vi "FastOffset.vi"() -> ()   [LabVIEW 2011]
panel:
  out "OffDEC_dir":string
  in  "Offset RA":dbl=-30.0 caption="A.D." format="%.2f"
  in  "Offset DEC":dbl caption="DEC" format="%.2f"
  out "OffRA_dir":string
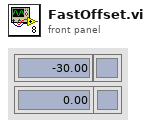
[diagram p1: front panel]
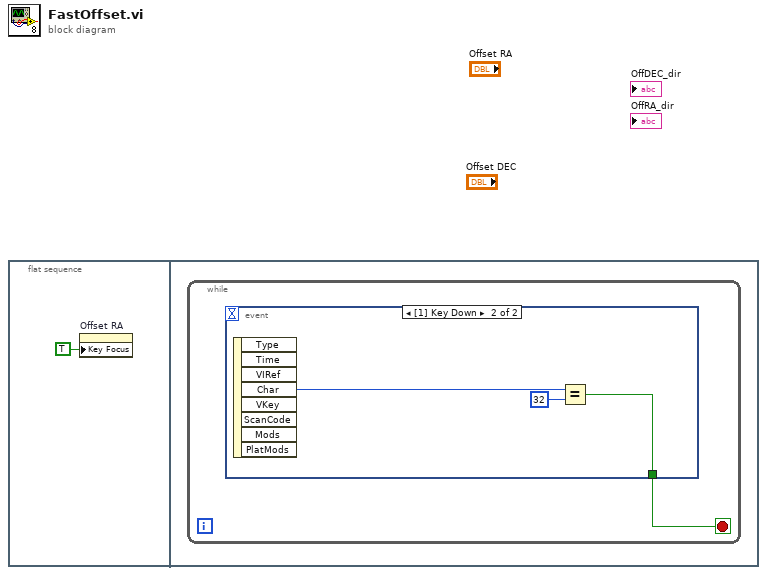
[diagram p0: block diagram]
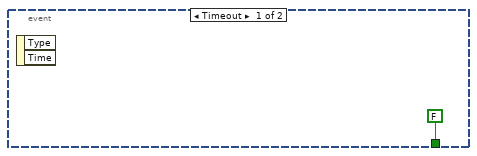
[diagram p2: hidden frame]
diagram:
  n1 = flat-sequence {
    frame #0 {
      n2 = property on="Offset RA" class="DigNum (strict)"("Key Focus"=TRUE) -> ()  [unwired: 2 in, 2 out]
    }
    frame #1 {
      n3 = while {
        stop <- w2 stop-if-true
        n4 = event shown="[1] Key Down" {
          selector: _ -> [_ _]
          dyn-events: _ -> [_ _]
          timeout: _ -> [_ _]
          tunnel: [FALSE w4] -> w2
          event Timeout {
            n5 = event-data() -> ()  [unwired: 1 in, 2 out]
          }
          event Key Down {
            n6 = event-data() -> ("Char"=w6:i16)  [unwired: 1 in, 7 out]
            n7 = Equal?(x=w6, y=i16 32) -> (x = y?=w4:bool)
          }
        }
      }
    }
  }
